vi "Get Index.vi"(8 "error in (no error)":errorcluster, 11 "Device in":refnum<class "Device.lvclass">) -> (0 "error out":errorcluster, 2 "Index":u32, 3 "Device out":refnum<class "Device.lvclass">)   [LabVIEW 2020, in "RTL-SDR.lvlib" / "Device.lvclass"]
uses:
  Device.lvclass
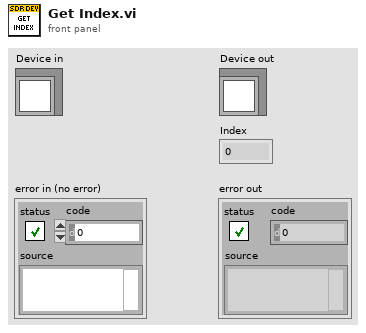
[diagram p1: front panel]
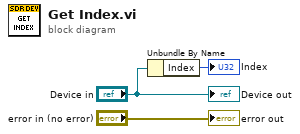
[diagram p0: block diagram]
diagram:
  n1 = Unbundle By Name("Device in") -> ("Index"=→"Index":u32)
  "error out" <- "error in (no error)"
  "Device out" <- "Device in"
